vi "graph.vi"() -> ()   [LabVIEW 2017]
panel:
  out "Waveform Graph 2":dbl[][](graph)
  out "Waveform Graph":dbl[][](graph)
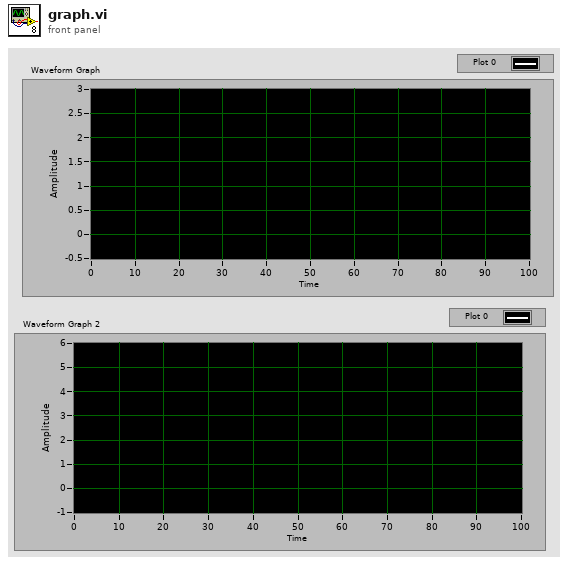
[diagram p1: front panel]
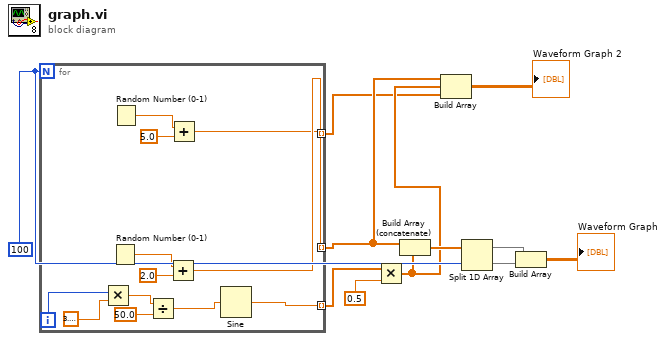
[diagram p0: block diagram]
diagram:
  w8 = 100
  n1 = for {
    N: w8 -> [_]
    tunnel: [w16] -> w4 mode=indexing
    tunnel: [w15] -> w11 mode=indexing
    tunnel: [w12] -> w1 mode=indexing
    i -> [w22]
    n2 = Multiply(x=w22, y=3.141592653589793) -> (x*y=w21:dbl)
    n3 = Random Number (0-1)() -> (number: 0 to 1=w18:dbl)
    n4 = Random Number (0-1)() -> (number: 0 to 1=w13:dbl)
    n5 = Divide(x=w21, y=50.0) -> (x/y=w19:dbl)
    n6 = Add(x=w18, y=2.0) -> (x+y=w16:dbl)
    n7 = Add(x=w13, y=5.0) -> (x+y=w12:dbl)
    n8 = Sine(x=w19) -> (sin(x)=w15:dbl)
  }
  n9 = Multiply(x=w11, y=0.5) -> (x*y=w3:dbl[])
  n10 = Build Array (concatenate)(w4, w3) -> (w9:dbl[])
  n11 = Build Array(w4, w3, w1) -> (→"Waveform Graph 2":dbl[][])
  n12 = Split 1D Array(array=w9, index=w8) -> (first subarray=w7:dbl[], second subarray=w6:dbl[])
  n13 = Build Array(w7, w6) -> (→"Waveform Graph":dbl[][])
